vi "Query Test Results.vi"() -> ()   [LabVIEW 2020]
uses:
  <vilib>/Skyline/Configuration/Configuration HTTP_class/NI Skyline Configuration HTTP.lvclass/NI Skyline Configuration HTTP.ctl
  <vilib>/Skyline/Configuration/Configuration HTTP_class/Open Configuration HTTP Auto.vi
  <vilib>/Skyline/Configuration/HTTP/Open Configuration Auto (Custom).vi
  <vilib>/Skyline/Configuration/HTTP/Configuration File Cache.vi
  <vilib>/Skyline/Configuration/HTTP/Initialize From Auto Configuration.vi
  <vilib>/httpClient/POSTBuffer.vi
  <vilib>/Skyline/Configuration/Configuration HTTP_class/NI Skyline Configuration HTTP.lvclass
  <vilib>/Skyline/Configuration/Configuration_class/NI Skyline Configuration.lvclass
  <vilib>/httpClient/LabVIEWHTTPClient.lvlib
panel:
  out "Status":string
  out "Started At":string
  out "System":string
  out "Results":i32
  in  "Serial Number":string
  in  "Part Number":string
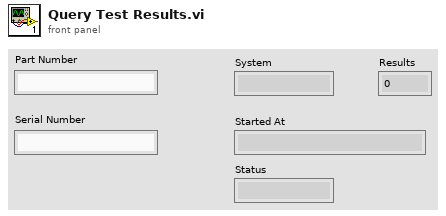
[diagram p1: front panel]
types:
  T1 = typedef "LabVIEWHTTPClient.lvlib/ClientHandle.ctl" = refnum<k1>
  T2 = cluster{"totalCount":i32, "continuationToken":string, "results":cluster{"status":cluster{"statusType":string, "statusName":string}, "serialNumber":string, "partNumber":string, "operator":string, "hostName":string, "startedAt":string}[]}
  T3 = cluster{"status":cluster{"statusType":string, "statusName":string}, "serialNumber":string, "partNumber":string, "operator":string, "hostName":string, "startedAt":string}[]
  T4 = cluster{"status":cluster{"statusType":string, "statusName":string}, "serialNumber":string, "partNumber":string, "operator":string, "hostName":string, "startedAt":string}
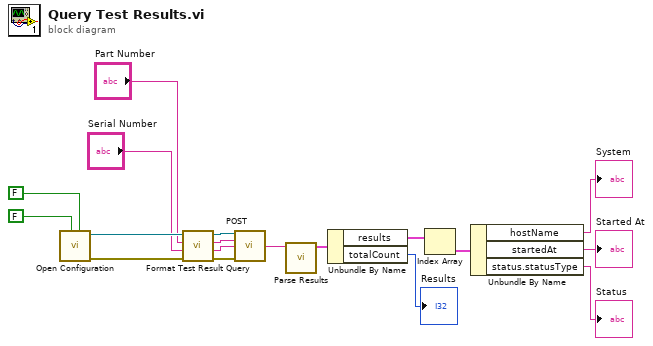
[diagram p0: block diagram]
diagram:
  n1 = call-poly <vilib>:"Open Configuration.vi"("HTTPS only?"=FALSE, "verify server?"=FALSE) -> ("error out"=w14:errorcluster, "configuration"=w15:refnum<class "NI Skyline Configuration HTTP.lvclass">)  [unwired: 8 in]
  n2 = call "Format Test Result Query.vi"("error in (no error)"=w14, "Serial Number"="Serial Number", "Part Number"="Part Number", "NI Skyline Configuration HTTP in"=w15) -> ("error out"=w13:errorcluster, "String"=w11:string, "String 2"=w12:string, "http session"=w16:T1)  [unwired: 4 in]
  n3 = call-poly <vilib>:"POST.vi"("client handle"=w16, "url"=w12, "buffer"=w11, "error in (no error)"=w13) -> ("body"=w8:string)  [unwired: 8 in, 3 out]
  n4 = call "Parse Results.vi"("body"=w8) -> ("test results"=w7:T2)  [unwired: 10 in]
  n5 = Unbundle By Name(w7) -> ("results"=w5:T3, "totalCount"=→"Results":i32)
  n6 = Index Array(array=w5) -> (element=w4:T4)  [unwired: 1 in]
  n7 = Unbundle By Name(w4) -> ("hostName"=→"System":string, "startedAt"=→"Started At":string, "status.statusType"=→"Status":string)
